vi "Handle Events.vi"(8 "error in (no error)":errorcluster, 11 "MulticolumnListboxEventHandler":refnum<class "MulticolumnListboxEventHandler.lvclass">) -> ()   [LabVIEW 2017, in "ActorEvents.lvlib" / "MulticolumnListboxEventHandler.lvclass"]
uses:
  MulticolumnListboxEventHandler.lvclass
  C:/Git/mva-framework/Framework/ActorEvents/IEventHandler/IEventHandler.lvclass
  MulticolumnListboxEventHandler.lvclass/MulticolumnListboxEventHandler.ctl
  IEventHandler/IEventHandler.lvclass/IEventHandler.ctl
  <vilib>/ActorFramework/Message Enqueuer/Message Enqueuer.lvclass/Message Enqueuer.ctl
  IEventAggregator Messages/EventDataMessage/EventDataMessage.lvclass/EventDataMessage.ctl
  IEventAggregator Messages/ControlDragSourceUpdateMsg/ControlDragSourceUpdateMsg.lvclass/ControlDragSourceUpdateMsg.ctl
  IEventAggregator Messages/ControlDragStartingMsg/ControlDragStartingMsg.lvclass/ControlDragStartingMsg.ctl
  IEventAggregator Messages/ControlMouseDownMsg/ControlMouseDownMsg.lvclass/ControlMouseDownMsg.ctl
  IEventAggregator Messages/ControlKeyDownMsg/ControlKeyDownMsg.lvclass/ControlKeyDownMsg.ctl
  IEventAggregator Messages/ListboxEditCellMsg/ListboxEditCellMsg.lvclass/ListboxEditCellMsg.ctl
  <vilib>/event_ctls.llb/lveventtype.ctl
  IEventAggregator Messages/EventDataMessage/Read Discarded.vi
  IEventAggregator Messages/ControlDragSourceUpdateMsg/Accessors/Read Cursor.vi
  IEventAggregator Messages/ControlDragStartingMsg/Accessors/Read Data.vi
  IEventAggregator Messages/ControlDragStartingMsg/Accessors/Read Drag Mode.vi
  IEventAggregator Messages/ControlMouseDownMsg/Accessors/Read Button.vi
  IEventAggregator Messages/ControlMouseDownMsg/Accessors/Read Mods.vi
  IEventAggregator Messages/ControlMouseDownMsg/Accessors/Read PlatMods.vi
  IEventAggregator Messages/ControlKeyDownMsg/Accessors/Read Char.vi
  IEventAggregator Messages/ControlKeyDownMsg/Accessors/Read VKey.vi
  IEventAggregator Messages/ControlKeyDownMsg/Accessors/Read Mods.vi
  IEventAggregator Messages/ControlKeyDownMsg/Accessors/Read PlatMods.vi
  IEventAggregator Messages/ControlKeyDownMsg/Accessors/Read FocusObj.vi
  IEventAggregator Messages/ListboxEditCellMsg/Accessors/Read String.vi
  IEventHandler/Accessors/Read Timeout [ms].vi
  IEventHandler/Accessors/Read Event Filter.vi
  IEventHandler/Accessors/Read EventAggregator Enqueuer.vi
  IEventHandler/Accessors/Read Timeout Message.vi
  IEventHandler/Accessors/Read Timeout Message Priority.vi
  IEventAggregator Messages/ControlDropMsg/ControlDropMsg.lvclass
  C:/Git/mva-framework/Framework/ActorEvents/IEventAggregator Messages/EventDataMessage/EventDataMessage.lvclass
  IEventAggregator Messages/ControlDragOverMsg/ControlDragOverMsg.lvclass
  IEventAggregator Messages/ControlDragSourceUpdateMsg/ControlDragSourceUpdateMsg.lvclass
  IEventAggregator Messages/ControlDragStartingMsg/ControlDragStartingMsg.lvclass
  IEventAggregator Messages/ControlMouseDownMsg/ControlMouseDownMsg.lvclass
  IEventAggregator Messages/ControlKeyDownMsg/ControlKeyDownMsg.lvclass
  IEventAggregator Messages/ListboxEditCellMsg/ListboxEditCellMsg.lvclass
  IEventAggregator Messages/ShortcutMenuActivationMsg/ShortcutMenuActivationMsg.lvclass
  IEventAggregator Messages/ShortcutMenuSelectionMsg/ShortcutMenuSelectionMsg.lvclass
  <vilib>/ActorFramework/Message Priority Queue/Priority Enqueue.vi
  <vilib>/ActorFramework/Message/Message.lvclass
  <vilib>/ActorFramework/Message Enqueuer/Message Enqueuer.lvclass
  IEventFilter/IEventFilter.lvclass
  IEventAggregator Messages/ValueChangeMsg/ValueChangeMsg.lvclass
  IEventAggregator Messages/ControlMouseUpMsg/ControlMouseUpMsg.lvclass
  IEventAggregator Messages/ListboxDoubleClickMsg/ListboxDoubleClickMsg.lvclass
  IEventAggregator Messages/ControlMouseEnterMsg/ControlMouseEnterMsg.lvclass
  IEventAggregator Messages/ControlMouseLeaveMsg/ControlMouseLeaveMsg.lvclass
  IEventAggregator Messages/ControlKeyUpMsg/ControlKeyUpMsg.lvclass
  IEventAggregator Messages/ControlDragEndedMsg/ControlDragEndedMsg.lvclass
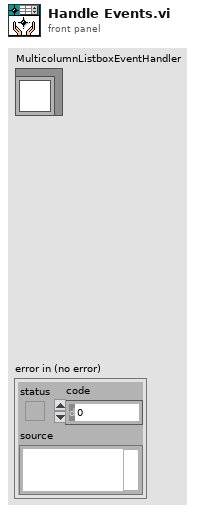
[diagram p1: front panel]
types:
  T1 = typedef "ActorEvents.lvlib/IEventFilter.lvclass/EventFilter Reference.ctl" = refnum<data-value>
  T2 = typedef "Actor Framework.lvlib/Message Enqueuer.lvclass/Message Priority.ctl" = enum16{"Low", "Normal", "High"}
  T3 = typedef "lveventtype.ctl" = enum32{"Null", "Timeout", "Annotation Menu Selection", "Annotation Menu Selection?", "App Instance Close", "App Instance Close?", "Autoscale Range Change", "Bookmark Info Change", "Cell Edit", "Cell Edit?", "Cursor Grab", "Cursor Grab?", "Cursor Menu Selection", "Cursor Menu Selection?", "Cursor Move", "Cursor Release", "Data Change", "Direction Change", "Display State Change", "Drag Ended", "Drag Enter", "Drag Leave", "Drag Over", "Drag Source Update", "Drag Starting", "Drag Starting?", "Drop", "Exec State Change", "Key Down", "Key Down?", "Key Repeat", "Key Repeat?", "Key Up", "Listbox Double Click", "Menu Activation?", "Menu Selection (App)", "Menu Selection? (App)", "Menu Selection (User)", "Mouse Down", "Mouse Down?", "Mouse Enter", "Mouse Leave", "Mouse Move", "Mouse Up", "Mouse Wheel", "NI Security User Change (App)", "Pane Size", "Panel Close", "Panel Close?", "Panel Resize", "Plot Attribute Change", "Scale Range Change", "Shortcut Menu Activation?", "Shortcut Menu Selection (App)", "Shortcut Menu Selection? (App)", "Shortcut Menu Selection (User)", "Tree Double Click", "Tree Drag", "Tree Drag?", "Tree Drop", "Tree Drop?", "Tree Item Close", "Tree Item Close?", "Tree Item Open", "Tree Item Open?", "User Event", "Value Change"}
  T4 = typedef "LVPoint32TypeDef.ctl" = cluster{"Horizontal":i32, "Vertical":i32}
  T5 = cluster{"Shift":bool, "Ctrl":bool, "Alt":bool, "Cmd":bool, "Opt":bool}
  T6 = cluster{"data name":string, "drag data":variant}[]
  T7 = typedef "eventvkey.ctl" = enum16{"ASCII", "Enter", "Return", "Shift", "Ctrl", "Alt", "Cmd", "Opt", "Caps", "NumLock", "Clear", "Break", "Up", "Down", "Left", "Right", "Insert", "Delete", "Home", "End", "PageUp", "PageDown", "Escape", "Help", "Pause", "ScrollLock", "F1", "F2", "F3", "F4", "F5", "F6", "F7", "F8", "F9", "F10", "F11", "F12", "F13", "F14", "F15", "F16", "F17", "F18", "F19", "F20", "F21", "F22", "F23", "F24", "Play", "VolumeUp", "VolumeDown", "Mute", "Two Byte Char"}
  T8 = typedef "LVRowAndColumnTypeDef.ctl" = cluster{"Row":i32, "Column":i32}
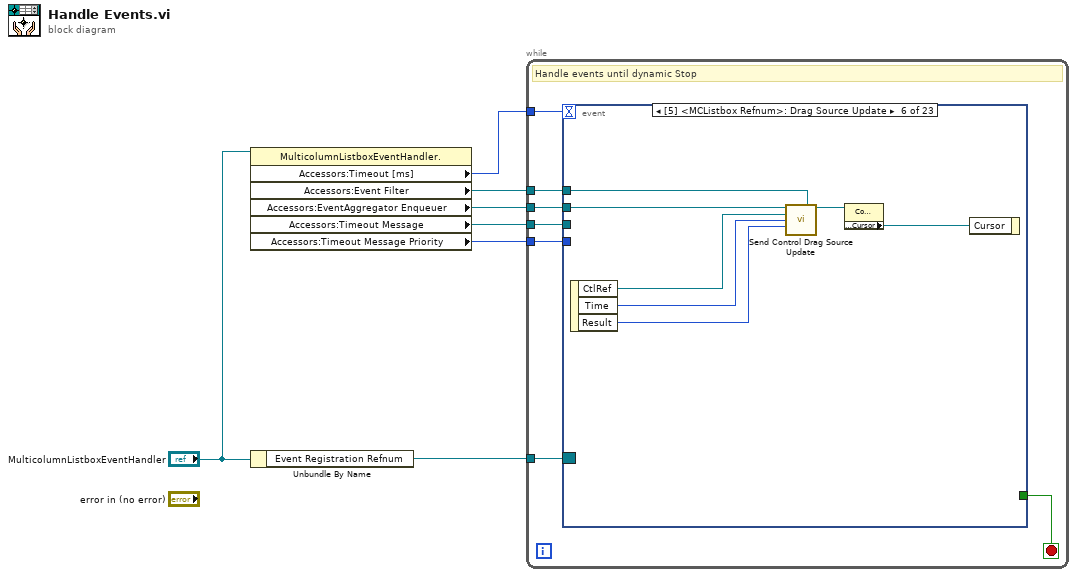
[diagram p0: block diagram]
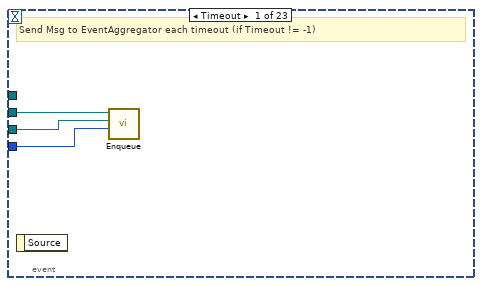
[diagram p2: hidden frame]
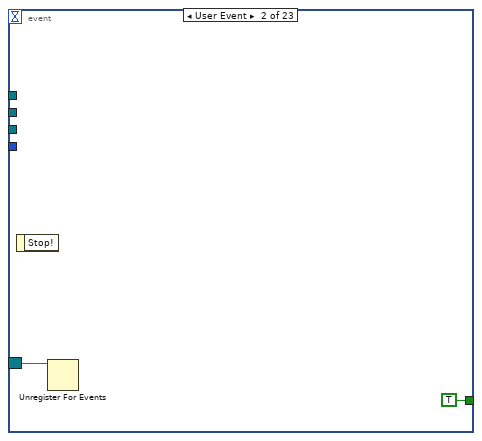
[diagram p3: hidden frame]
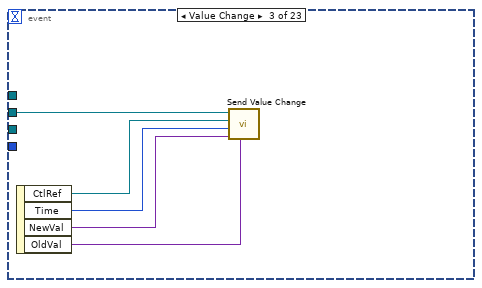
[diagram p4: hidden frame]
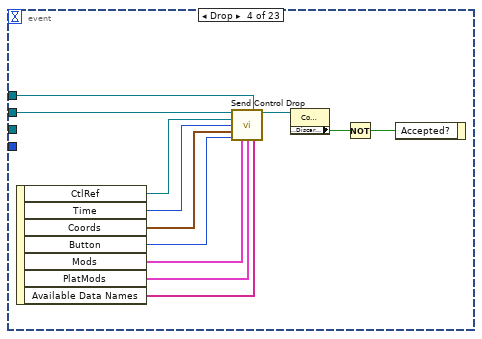
[diagram p5: hidden frame]
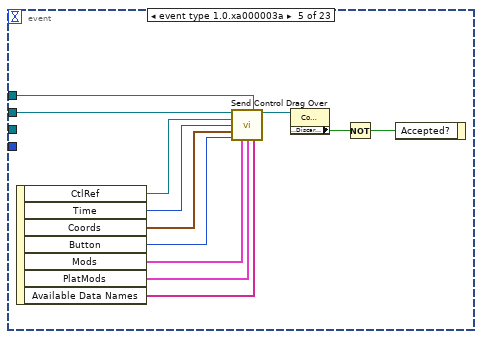
[diagram p6: hidden frame]
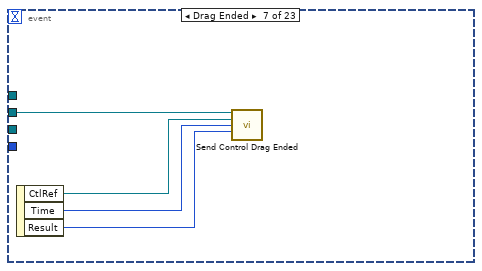
[diagram p7: hidden frame]
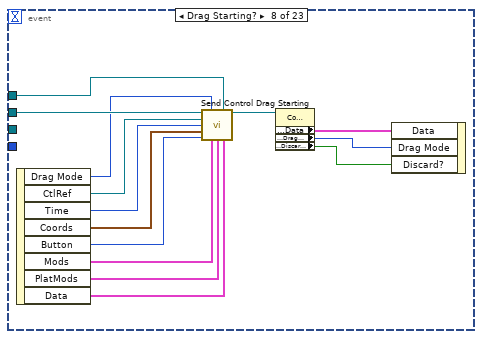
[diagram p8: hidden frame]
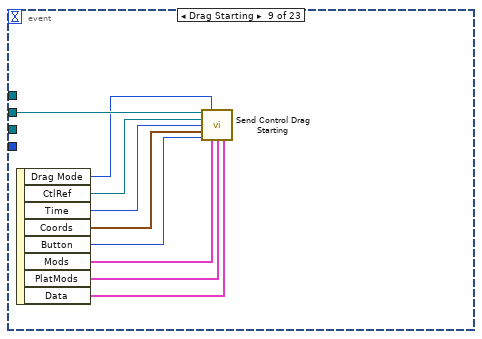
[diagram p9: hidden frame]
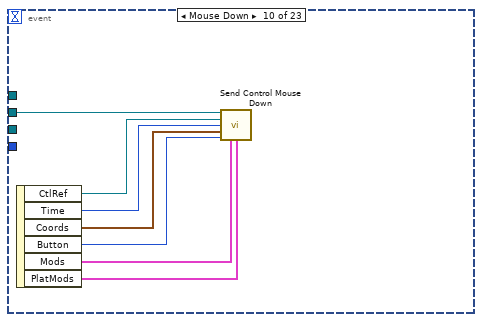
[diagram p10: hidden frame]
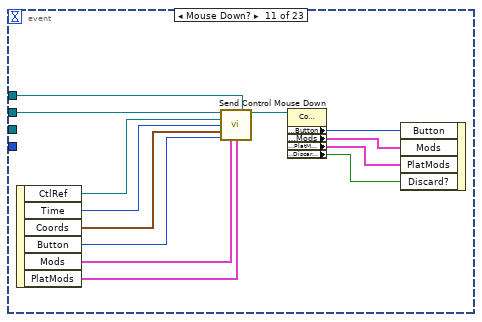
[diagram p11: hidden frame]
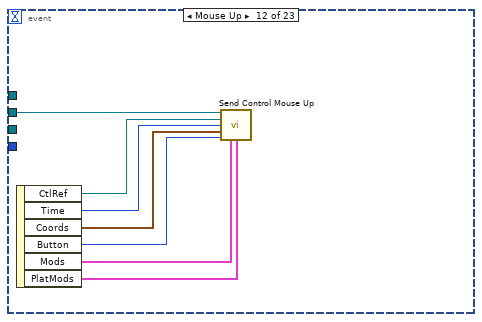
[diagram p12: hidden frame]
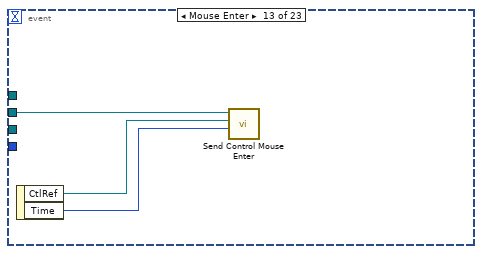
[diagram p13: hidden frame]
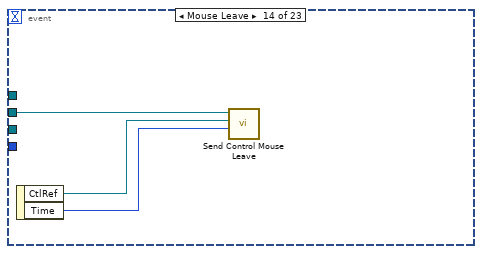
[diagram p14: hidden frame]
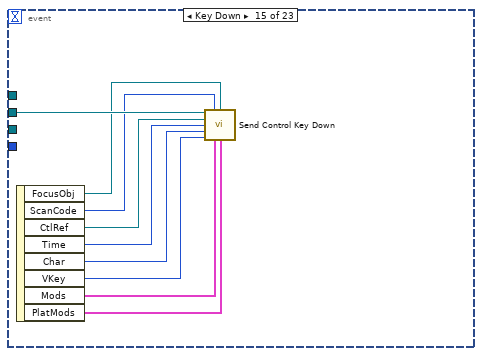
[diagram p15: hidden frame]
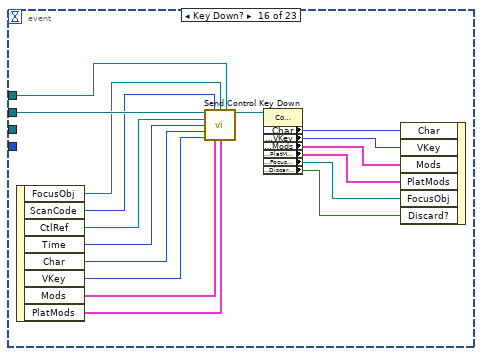
[diagram p16: hidden frame]
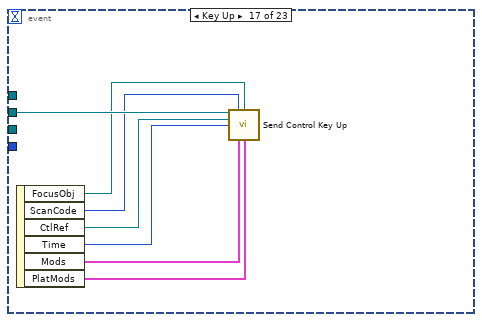
[diagram p17: hidden frame]
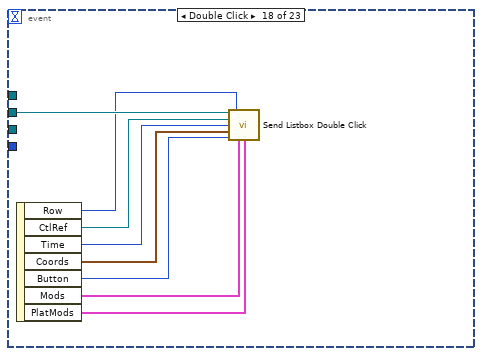
[diagram p18: hidden frame]
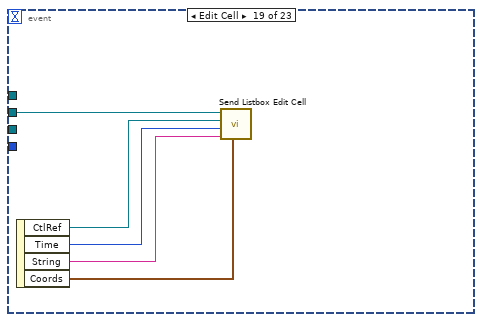
[diagram p19: hidden frame]
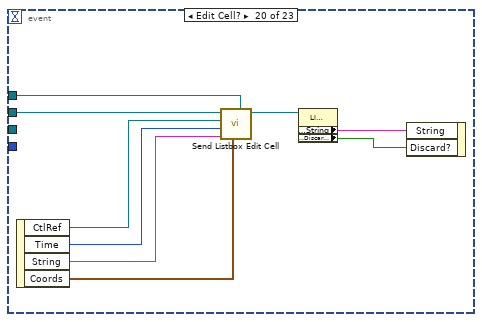
[diagram p20: hidden frame]
diagram:
  n1 = property class="MulticolumnListboxEventHandler."(reference="MulticolumnListboxEventHandler") -> ("Accessors:Timeout [ms]"=w5:i32, "Accessors:Event Filter"=w3:T1, "Accessors:EventAggregator Enqueuer"=w4:refnum<class "Message Enqueuer.lvclass">, "Accessors:Timeout Message"=w2:refnum<class "Message.lvclass">, "Accessors:Timeout Message Priority"=w1:T2)  [unwired: 1 in, 2 out]
  n2 = Unbundle By Name("MulticolumnListboxEventHandler") -> ("Event Registration Refnum"=w7:refnum<event-registration>)
  n3 = while {
    tunnel: w7 -> [w14]
    tunnel: w4 -> [w13]
    tunnel: w2 -> [w12]
    tunnel: w1 -> [w11]
    tunnel: w5 -> [w10]
    tunnel: w3 -> [w8]
    stop <- w9 stop-if-true
    # "Handle events until dynamic Stop"
    n4 = event shown="[5] <MCListbox Refnum>: Drag Source Update" {
      selector: w14 -> [_ w19 _ _ _ _ _ _ _ _ _ _ _ _ _ _ _ _ _ _ _ _ _]
      dyn-events: _ -> [_ _ _ _ _ _ _ _ _ _ _ _ _ _ _ _ _ _ _ _ _ _ _]
      timeout: w10 -> [_ _ _ _ _ _ _ _ _ _ _ _ _ _ _ _ _ _ _ _ _ _ _]
      tunnel: [_ TRUE ("Stop!") _ _ _ _ _ _ _ _ _ _ _ _ _ _ _ _ _ _ _ _ _] -> w9
      tunnel: w13 -> [w17 _ w24 w34 w46 w54 w59 w73 w82 w89 w102 w109 w112 w115 w124 w141 w148 w156 w161 w170 w179 w189 w200]
      tunnel: w12 -> [w16 _ _ _ _ _ _ _ _ _ _ _ _ _ _ _ _ _ _ _ _ _ _]
      tunnel: w11 -> [w15 _ _ _ _ _ _ _ _ _ _ _ _ _ _ _ _ _ _ _ _ _ _]
      tunnel: w8 -> [_ _ _ w25 w37 w51 _ w64 _ _ w95 _ _ _ _ w132 _ _ _ w165 w173 _ w193]
      event Timeout {
        # "Send Msg to EventAggregator each timeout (if Timeout != -1)"
        n5 = event-data() -> ()  [unwired: 1 in, 1 out]
        n6 = call <vilib>:"Enqueue.vi"("Message Priority (Normal)"=w15, "Message"=w16, "Message Enqueuer in"=w17) -> ()  [unwired: 7 in, 2 out]
      }
      event User Event {
        n7 = event-data() -> ()  [unwired: 1 in, 1 out]
        n8 = Unregister For Events(event registration refnum=w19) -> ()  [unwired: 1 in, 1 out]
      }
      event Value Change {
        n9 = event-data() -> ("CtlRef"=w21:refnum<vi>, "Time"=w23:u32, "NewVal"=w22:variant, "OldVal"=w20:variant)  [unwired: 1 in]
        n10 = call "Send Value Change.vi"("Old Value"=w20, "New Value"=w22, "Time"=w23, "Ctl Refnum"=w21, "Message Enqueuer in"=w24) -> ()  [unwired: 6 in, 1 out]
      }
      event Drop {
        n11 = event-data() -> ("CtlRef"=w32:refnum<vi>, "Time"=w31:u32, "Coords"=w30:T4, "Button"=w29:u16, "Mods"=w28:cluster{"Double Click":bool, "Menu Key":bool}, "PlatMods"=w27:T5, "Available Data Names"=w26:string[])  [unwired: 1 in]
        n12 = call "Send Control Drop.vi"("Message Enqueuer in"=w34, "EventFilter Reference"=w25, "CtlRef"=w32, "Time"=w31, "Coords"=w30, "Button"=w29, "Mods"=w28, "PlatMods"=w27, "Available Data Names"=w26) -> ("Filtered EventDataMessage"=w36:refnum<class "ControlDropMsg.lvclass">)  [unwired: 5 in, 1 out]
        n13 = property class="ControlDropMsg.lvclass"(reference=w36) -> ("Accessors:Discarded?"=w35:bool)  [unwired: 1 in, 2 out]
        n14 = Not(x=w35) -> (.not. x?=w33:bool)
        n15 = event-data("Accepted?"=w33) -> ()  [unwired: 1 in, 1 out]
      }
      event event type 1.0.xa000003a {
        n16 = event-data() -> ("CtlRef"=w44:refnum<vi>, "Time"=w43:u32, "Coords"=w42:T4, "Button"=w41:u16, "Mods"=w40:cluster{"Double Click":bool, "Menu Key":bool}, "PlatMods"=w39:T5, "Available Data Names"=w38:string[])  [unwired: 1 in]
        n17 = call "Send Control Drag Over.vi"("Message Enqueuer in"=w46, "EventFilter Reference"=w37, "CtlRef"=w44, "Time"=w43, "Coords"=w42, "Button"=w41, "Mods"=w40, "PlatMods"=w39, "Available Data Names"=w38) -> ("Filtered EventDataMessage"=w48:refnum<class "ControlDragOverMsg.lvclass">)  [unwired: 5 in, 1 out]
        n18 = property class="ControlDragOverMsg.lvclass"(reference=w48) -> ("Accessors:Discarded?"=w47:bool)  [unwired: 1 in, 2 out]
        n19 = Not(x=w47) -> (.not. x?=w45:bool)
        n20 = event-data("Accepted?"=w45) -> ()  [unwired: 1 in, 1 out]
      }
      event Drag Source Update {
        n21 = event-data() -> ("CtlRef"=w53:refnum<vi>, "Time"=w52:u32, "Result"=w49:enum16{"Drop Cancel", "Drop Move", "Drop Copy"})  [unwired: 1 in]
        n22 = call "Send Control Drag Source Update.vi"("Message Enqueuer in"=w54, "EventFilter Reference"=w51, "CtlRef"=w53, "Time"=w52, "Result"=w49) -> ("Filtered EventDataMessage"=w55:refnum<class "ControlDragSourceUpdateMsg.lvclass">)  [unwired: 9 in, 1 out]
        n23 = property class="ControlDragSourceUpdateMsg.lvcl"(reference=w55) -> ("Accessors:Cursor"=w50:refnum<k1>)  [unwired: 1 in, 2 out]
        n24 = event-data("Cursor"=w50) -> ()  [unwired: 1 in, 1 out]
      }
      event Drag Ended {
        n25 = event-data() -> ("CtlRef"=w58:refnum<vi>, "Time"=w57:u32, "Result"=w56:enum16{"Drop Cancel", "Drop Move", "Drop Copy"})  [unwired: 1 in]
        n26 = call "Send Control Drag Ended.vi"("Message Enqueuer in"=w59, "CtlRef"=w58, "Time"=w57, "Result"=w56) -> ()  [unwired: 10 in, 2 out]
      }
      event Drag Starting? {
        n27 = event-data() -> ("Drag Mode"=w65:enum32{"copy or move", "copy only", "move only"}, "CtlRef"=w72:refnum<vi>, "Time"=w71:u32, "Coords"=w70:T4, "Button"=w69:u16, "Mods"=w68:cluster{"Double Click":bool, "Menu Key":bool}, "PlatMods"=w67:T5, "Data"=w66:T6)  [unwired: 1 in]
        n28 = call "Send Control Drag Starting.vi"("Message Enqueuer in"=w73, "Drag Mode"=w65, "EventFilter Reference"=w64, "CtlRef"=w72, "Time"=w71, "Coords"=w70, "Button"=w69, "Mods"=w68, "PlatMods"=w67, "Data"=w66) -> ("Filtered EventDataMessage"=w63:refnum<class "ControlDragStartingMsg.lvclass">)  [unwired: 4 in, 1 out]
        n29 = property class="ControlDragStartingMsg.lvclass"(reference=w63) -> ("Accessors:Data"=w61:T6, "Accessors:Drag Mode"=w60:enum32{"copy or move", "copy only", "move only"}, "Accessors:Discarded?"=w62:bool)  [unwired: 1 in, 2 out]
        n30 = event-data("Data"=w61, "Drag Mode"=w60, "Discard?"=w62) -> ()  [unwired: 1 in, 1 out]
      }
      event Drag Starting {
        n31 = event-data() -> ("Drag Mode"=w74:enum32{"copy or move", "copy only", "move only"}, "CtlRef"=w81:refnum<vi>, "Time"=w80:u32, "Coords"=w79:T4, "Button"=w78:u16, "Mods"=w77:cluster{"Double Click":bool, "Menu Key":bool}, "PlatMods"=w76:T5, "Data"=w75:T6)  [unwired: 1 in]
        n32 = call "Send Control Drag Starting.vi"("Message Enqueuer in"=w82, "Drag Mode"=w74, "CtlRef"=w81, "Time"=w80, "Coords"=w79, "Button"=w78, "Mods"=w77, "PlatMods"=w76, "Data"=w75) -> ()  [unwired: 5 in, 2 out]
      }
      event Mouse Down {
        n33 = event-data() -> ("CtlRef"=w88:refnum<vi>, "Time"=w87:u32, "Coords"=w86:T4, "Button"=w85:u16, "Mods"=w84:cluster{"Double Click":bool, "Menu Key":bool}, "PlatMods"=w83:T5)  [unwired: 1 in]
        n34 = call "Send Control Mouse Down.vi"("Message Enqueuer in"=w89, "Ctl Refnum"=w88, "Time"=w87, "Coords"=w86, "Button"=w85, "Mods"=w84, "PlatMods"=w83) -> ()  [unwired: 7 in, 2 out]
      }
      event Mouse Down? {
        n35 = event-data() -> ("CtlRef"=w101:refnum<vi>, "Time"=w100:u32, "Coords"=w99:T4, "Button"=w98:u16, "Mods"=w97:cluster{"Double Click":bool, "Menu Key":bool}, "PlatMods"=w96:T5)  [unwired: 1 in]
        n36 = call "Send Control Mouse Down.vi"("Message Enqueuer in"=w102, "EventFilter Reference"=w95, "Ctl Refnum"=w101, "Time"=w100, "Coords"=w99, "Button"=w98, "Mods"=w97, "PlatMods"=w96) -> ("Filtered EventDataMessage"=w94:refnum<class "ControlMouseDownMsg.lvclass">)  [unwired: 6 in, 1 out]
        n37 = property class="ControlMouseDownMsg.lvclass"(reference=w94) -> ("Accessors:Button"=w93:u16, "Accessors:Mods"=w92:cluster{"Double Click":bool, "Menu Key":bool}, "Accessors:PlatMods"=w91:T5, "Accessors:Discarded?"=w90:bool)  [unwired: 1 in, 2 out]
        n38 = event-data("Button"=w93, "Mods"=w92, "PlatMods"=w91, "Discard?"=w90) -> ()  [unwired: 1 in, 1 out]
      }
      event Mouse Up {
        n39 = event-data() -> ("CtlRef"=w108:refnum<vi>, "Time"=w107:u32, "Coords"=w106:T4, "Button"=w105:u16, "Mods"=w104:cluster{"Double Click":bool, "Menu Key":bool}, "PlatMods"=w103:T5)  [unwired: 1 in]
        n40 = call "Send Control Mouse Up.vi"("Message Enqueuer in"=w109, "Ctl Refnum"=w108, "Time"=w107, "Coords"=w106, "Button"=w105, "Mods"=w104, "PlatMods"=w103) -> ()  [unwired: 8 in, 1 out]
      }
      event Mouse Enter {
        n41 = event-data() -> ("CtlRef"=w111:refnum<vi>, "Time"=w110:u32)  [unwired: 1 in]
        n42 = call "Send Control Mouse Enter.vi"("Time"=w110, "Ctl Refnum"=w111, "Message Enqueuer in"=w112) -> ()  [unwired: 8 in, 1 out]
      }
      event Mouse Leave {
        n43 = event-data() -> ("CtlRef"=w114:refnum<vi>, "Time"=w113:u32)  [unwired: 1 in]
        n44 = call "Send Control Mouse Leave.vi"("Time"=w113, "Ctl Refnum"=w114, "Message Enqueuer in"=w115) -> ()  [unwired: 8 in, 1 out]
      }
      event Key Down {
        n45 = event-data() -> ("FocusObj"=w123:refnum<vi>, "ScanCode"=w122:i16, "CtlRef"=w121:refnum<vi>, "Time"=w120:u32, "Char"=w119:i16, "VKey"=w118:T7, "Mods"=w117:cluster{"Num Pad":bool, "Menu Key":bool}, "PlatMods"=w116:T5)  [unwired: 1 in]
        n46 = call "Send Control Key Down.vi"("Message Enqueuer in"=w124, "ScanCode"=w122, "FocusObj"=w123, "CtlRef"=w121, "Time"=w120, "Char"=w119, "VKey"=w118, "Mods"=w117, "PlatMods"=w116) -> ()  [unwired: 5 in, 2 out]
      }
      event Key Down? {
        n47 = event-data() -> ("FocusObj"=w140:refnum<vi>, "ScanCode"=w139:i16, "CtlRef"=w138:refnum<vi>, "Time"=w137:u32, "Char"=w136:i16, "VKey"=w135:T7, "Mods"=w134:cluster{"Num Pad":bool, "Menu Key":bool}, "PlatMods"=w133:T5)  [unwired: 1 in]
        n48 = call "Send Control Key Down.vi"("Message Enqueuer in"=w141, "ScanCode"=w139, "FocusObj"=w140, "EventFilter Reference"=w132, "CtlRef"=w138, "Time"=w137, "Char"=w136, "VKey"=w135, "Mods"=w134, "PlatMods"=w133) -> ("Filtered EventDataMessage"=w131:refnum<class "ControlKeyDownMsg.lvclass">)  [unwired: 4 in, 1 out]
        n49 = property class="ControlKeyDownMsg.lvclass"(reference=w131) -> ("Accessors:Char"=w130:i16, "Accessors:VKey"=w129:T7, "Accessors:Mods"=w128:cluster{"Double Click":bool, "Menu Key":bool}, "Accessors:PlatMods"=w127:T5, "Accessors:FocusObj"=w126:refnum<vi>, "Accessors:Discarded?"=w125:bool)  [unwired: 1 in, 2 out]
        n50 = event-data("Char"=w130, "VKey"=w129, "Mods"=w128, "PlatMods"=w127, "FocusObj"=w126, "Discard?"=w125) -> ()  [unwired: 1 in, 1 out]
      }
      event Key Up {
        n51 = event-data() -> ("FocusObj"=w147:refnum<vi>, "ScanCode"=w146:i16, "CtlRef"=w145:refnum<vi>, "Time"=w144:u32, "Mods"=w143:cluster{"Num Pad":bool, "Menu Key":bool}, "PlatMods"=w142:T5)  [unwired: 1 in]
        n52 = call "Send Control Key Up.vi"("Message Enqueuer in"=w148, "ScanCode"=w146, "FocusObj"=w147, "Ctl Refnum"=w145, "Time"=w144, "Mods"=w143, "PlatMods"=w142) -> ()  [unwired: 8 in, 1 out]
      }
      event Double Click {
        n53 = event-data() -> ("Row"=w149:i32, "CtlRef"=w155:refnum<vi>, "Time"=w154:u32, "Coords"=w153:T4, "Button"=w152:u16, "Mods"=w151:cluster{"Double Click":bool, "Menu Key":bool}, "PlatMods"=w150:T5)  [unwired: 1 in]
        n54 = call "Send Listbox Double Click.vi"("Message Enqueuer in"=w156, "Row"=w149, "Ctl Refnum"=w155, "Time"=w154, "Coords"=w153, "Button"=w152, "Mods"=w151, "PlatMods"=w150) -> ()  [unwired: 7 in, 1 out]
      }
      event Edit Cell {
        n55 = event-data() -> ("CtlRef"=w160:refnum<vi>, "Time"=w159:u32, "String"=w158:string, "Coords"=w157:T8)  [unwired: 1 in]
        n56 = call "Send Listbox Edit Cell.vi"("Coords"=w157, "String"=w158, "Time"=w159, "CtlRef"=w160, "Message Enqueuer in"=w161) -> ()  [unwired: 5 in, 2 out]
      }
      event Edit Cell? {
        n57 = event-data() -> ("CtlRef"=w169:refnum<vi>, "Time"=w168:u32, "String"=w167:string, "Coords"=w166:T8)  [unwired: 1 in]
        n58 = call "Send Listbox Edit Cell.vi"("EventFilter Reference"=w165, "Coords"=w166, "String"=w167, "Time"=w168, "CtlRef"=w169, "Message Enqueuer in"=w170) -> ("Filtered EventDataMessage"=w164:refnum<class "ListboxEditCellMsg.lvclass">)  [unwired: 4 in, 1 out]
        n59 = property class="ListboxEditCellMsg.lvclass"(reference=w164) -> ("Accessors:String"=w163:string, "Accessors:Discarded?"=w162:bool)  [unwired: 1 in, 2 out]
        n60 = event-data("String"=w163, "Discard?"=w162) -> ()  [unwired: 1 in, 1 out]
      }
      event Shortcut Menu Activation? {
        n61 = event-data() -> ("CtlRef"=w174:refnum<vi>, "Time"=w178:u32, "MenuRef"=w175:refnum<k9>, "Coords"=w177:T4, "SubObj"=w176:refnum<vi>)  [unwired: 1 in]
        n62 = call "Send Shortcut Menu Activation.vi"("Message Enqueuer in"=w179, "EventFilter Reference"=w173, "CtlRef"=w174, "Time"=w178, "MenuRef"=w175, "Coords"=w177, "SubObj"=w176) -> ("Filtered EventDataMessage"=w172:refnum<class "ShortcutMenuActivationMsg.lvclass">)  [unwired: 7 in, 1 out]
        n63 = property class="ShortcutMenuActivationMsg.lvcla"(reference=w172) -> ("Accessors:Discarded?"=w171:bool)  [unwired: 1 in, 2 out]
        n64 = event-data("Discard?"=w171) -> ()  [unwired: 1 in, 1 out]
      }
      event Shortcut Menu Selection (User); Shortcut Menu Selection (App) {
        n65 = event-data() -> ("Type"=w182:T3, "CtlRef"=w188:refnum<vi>, "Time"=w187:u32, "ItemTag"=w186:string, "ItemPath"=w185:string, "Coords"=w184:T4, "SubObj"=w183:refnum<vi>)  [unwired: 1 in]
        n66 = Equal?(x=lveventtype."Shortcut Menu Selection (App)", y=w182) -> (x = y?=w181:bool)
        n67 = call "Send Shortcut Menu Selection.vi"("Message Enqueuer in"=w189, "App Item?"=w181, "CtlRef"=w188, "Time"=w187, "Item Tag"=w186, "Item Path"=w185, "Coords"=w184, "SubObj"=w183) -> ()  [unwired: 6 in, 2 out]
      }
      event Shortcut Menu Selection? (App) {
        w192 = TRUE  # App Item?
        n68 = event-data() -> ("CtlRef"=w199:refnum<vi>, "Time"=w198:u32, "ItemTag"=w197:string, "ItemPath"=w196:string, "Coords"=w195:T4, "SubObj"=w194:refnum<vi>)  [unwired: 1 in, 1 out]
        n69 = call "Send Shortcut Menu Selection.vi"("Message Enqueuer in"=w200, "App Item?"=w192, "EventFilter Reference"=w193, "CtlRef"=w199, "Time"=w198, "Item Tag"=w197, "Item Path"=w196, "Coords"=w195, "SubObj"=w194) -> ("Filtered EventDataMessage"=w191:refnum<class "ShortcutMenuSelectionMsg.lvclass">)  [unwired: 5 in, 1 out]
        n70 = property class="ShortcutMenuSelectionMsg.lvclas"(reference=w191) -> ("Accessors:Discarded?"=w190:bool)  [unwired: 1 in, 2 out]
        n71 = event-data("Discard?"=w190) -> ()  [unwired: 1 in, 1 out]
      }
    }
  }
